vi "Autonomous Independent.vi"   [LabVIEW 2015]
doc: "This VI is called when autonomous begins, and will automatically be terminated when autonomous ends. You can carry out timed or sensor driven robot movement independently without needing to return to the caller."
uses:
  <vilib>/Rock Robotics/WPI/Utilities/WPI_GetSetVariantRefNum.vi
  <vilib>/Rock Robotics/Network Tables/NT Read String.vi
  <vilib>/Rock Robotics/Network Tables/NT Read Number.vi
  <vilib>/Rock Robotics/Network Tables/NT Write Numeric Array.vi
  <vilib>/Rock Robotics/Network Tables/NT Read Boolean.vi
panel:
  # "Be sure to right-click and choose Data Operations>>Make Current Value default if you want to save the array values with the VI"
types:
  T1 = typedef "WPI_JoystickDevRef.ctl" = cluster{"Device":T2}
  T2 = typedef "WPI_JoystickDeviceEnum.ctl" = enum16{"USB 0", "USB 1", "USB 2", "USB 3", "USB 4", "USB 5"}
  T3 = typedef "WPI_EncoderDevRef.ctl" = cluster{"DevStatus":errorcluster, "EncoderIndex":T4, "CounterIndex":T5, "DistancePerCount":dbl, "Decoding Type":T6}
  T4 = typedef "FPGA_EncoderIdx.ctl" = enum8{"Enc 0", "Enc 1", "Enc 2", "Enc 3", "Enc 4", "Enc 5", "Enc 6", "Enc 7", "Invalid"}
  T5 = typedef "FPGA_CounterCtrSystemIndex.ctl" = enum8{"Ctr 0", "Ctr 1", "Ctr 2", "Ctr 3", "Ctr 4", "Ctr 5", "Ctr 6", "Ctr 7", "Invalid"}
  T6 = typedef "WPI_EncoderType.ctl" = enum16{"1x", "2x", "4x"}
  T7 = typedef "WPI_MotorControlDeviceRef.ctl" = cluster{"DeviceStatus":errorcluster, "Type":T8, "PWM":cluster{"PWM Channel":T9, "DeadBand":T10}, "CAN":cluster{"Device Number":u8, "Control Mode":T11, "Semaphore":T12, "Max Vout":dbl, "TalonSRX Control Mode":T13}, "Invert":bool}
  T8 = typedef "WPI_MotorControlType.ctl" = enum16{"PWM", "CAN", "CANTalonSRX"}
  T9 = typedef "FPGA_DIOPWMChannel.ctl" = enum8{"PWM 0", "PWM 1", "PWM 2", "PWM 3", "PWM 4", "PWM 5", "PWM 6", "PWM 7", "PWM 8", "PWM 9", "PWM MXP 0", "PWM MXP 1", "PWM MXP 2", "PWM MXP 3", "PWM MXP 4", "PWM MXP 5", "PWM MXP 6", "PWM MXP 7", "PWM MXP 8", "PWM MXP 9", "Invalid"}
  T10 = typedef "WPI_PWMDeadband.ctl" = cluster{"Name":string, "maxPositivePwm":i32, "minPositivePwm":i32, "centerPwm":i32, "maxNegativePwm":i32, "minNegativePwm":i32, "angularRange":u16}
  T11 = typedef "WPI_CANJaguar_ControlMode.ctl" = enum8{"Percent VBus", "Current", "Speed", "Position", "Voltage"}
  T12 = typedef "Semaphore RefNum" = refnum<k1>
  T13 = typedef "WPI_CANTalonSRX_APIControlMode.ctl" = enum8{"Percent VBus", "Speed", "Position", "Slave", "Unchanged / Invalid", "Voltage Compensation", "Current", "Motion Profile"}
  T14 = typedef "WPI_GyroDevRef.ctl" = cluster{"DevStatus":errorcluster, "Analog Channel":T15, "Offset":dbl, "Gain (VoltsPerDegree/Second)":dbl, "Gyro Type":enum16{"Analog", "XRS450"}, "Handle":i32, "SPI Bus":T16, "Device Found":bool, "Sample Rate":dbl, "Calibrate On Open":bool}
  T15 = typedef "FPGA_AIChannel.ctl" = enum8{"AI 0", "AI 1", "AI 2", "AI 3", "AI MXP 0", "AI MXP 1", "AI MXP 2", "AI MXP 3", "Invalid"}
  T16 = typedef "spi_bus.ctl" = enum16{"SPI On-Board, CS0", "SPI On-Board, CS1", "SPI On-Board, CS2", "SPI On-Board, CS3", "SPI MXP", "Invalid"}
  T17 = typedef "WPI_RobotDriveDevRef.ctl" = cluster{"DevStatus":errorcluster, "Motors[]":T7[], "Square Inputs":bool, "Max Output":dbl}
  T18 = typedef "WPI_DigitalInputDevRef.ctl" = cluster{"DevStatus":errorcluster, "DIO Channel":T19}
  T19 = typedef "FPGA_DIOChannel.ctl" = enum8{"DIO 0", "DIO 1", "DIO 2", "DIO 3", "DIO 4", "DIO 5", "DIO 6", "DIO 7", "DIO 8", "DIO 9", "DIO MXP 0", "DIO MXP 1", "DIO MXP 2", "DIO MXP 3", "DIO MXP 4", "DIO MXP 5", "DIO MXP 6", "DIO MXP 7", "DIO MXP 8", "DIO MXP 9", "DIO MXP 10", "DIO MXP 11", "DIO MXP 12", "DIO MXP 13", "DIO MXP 14", "DIO MXP 15", "Invalid"}
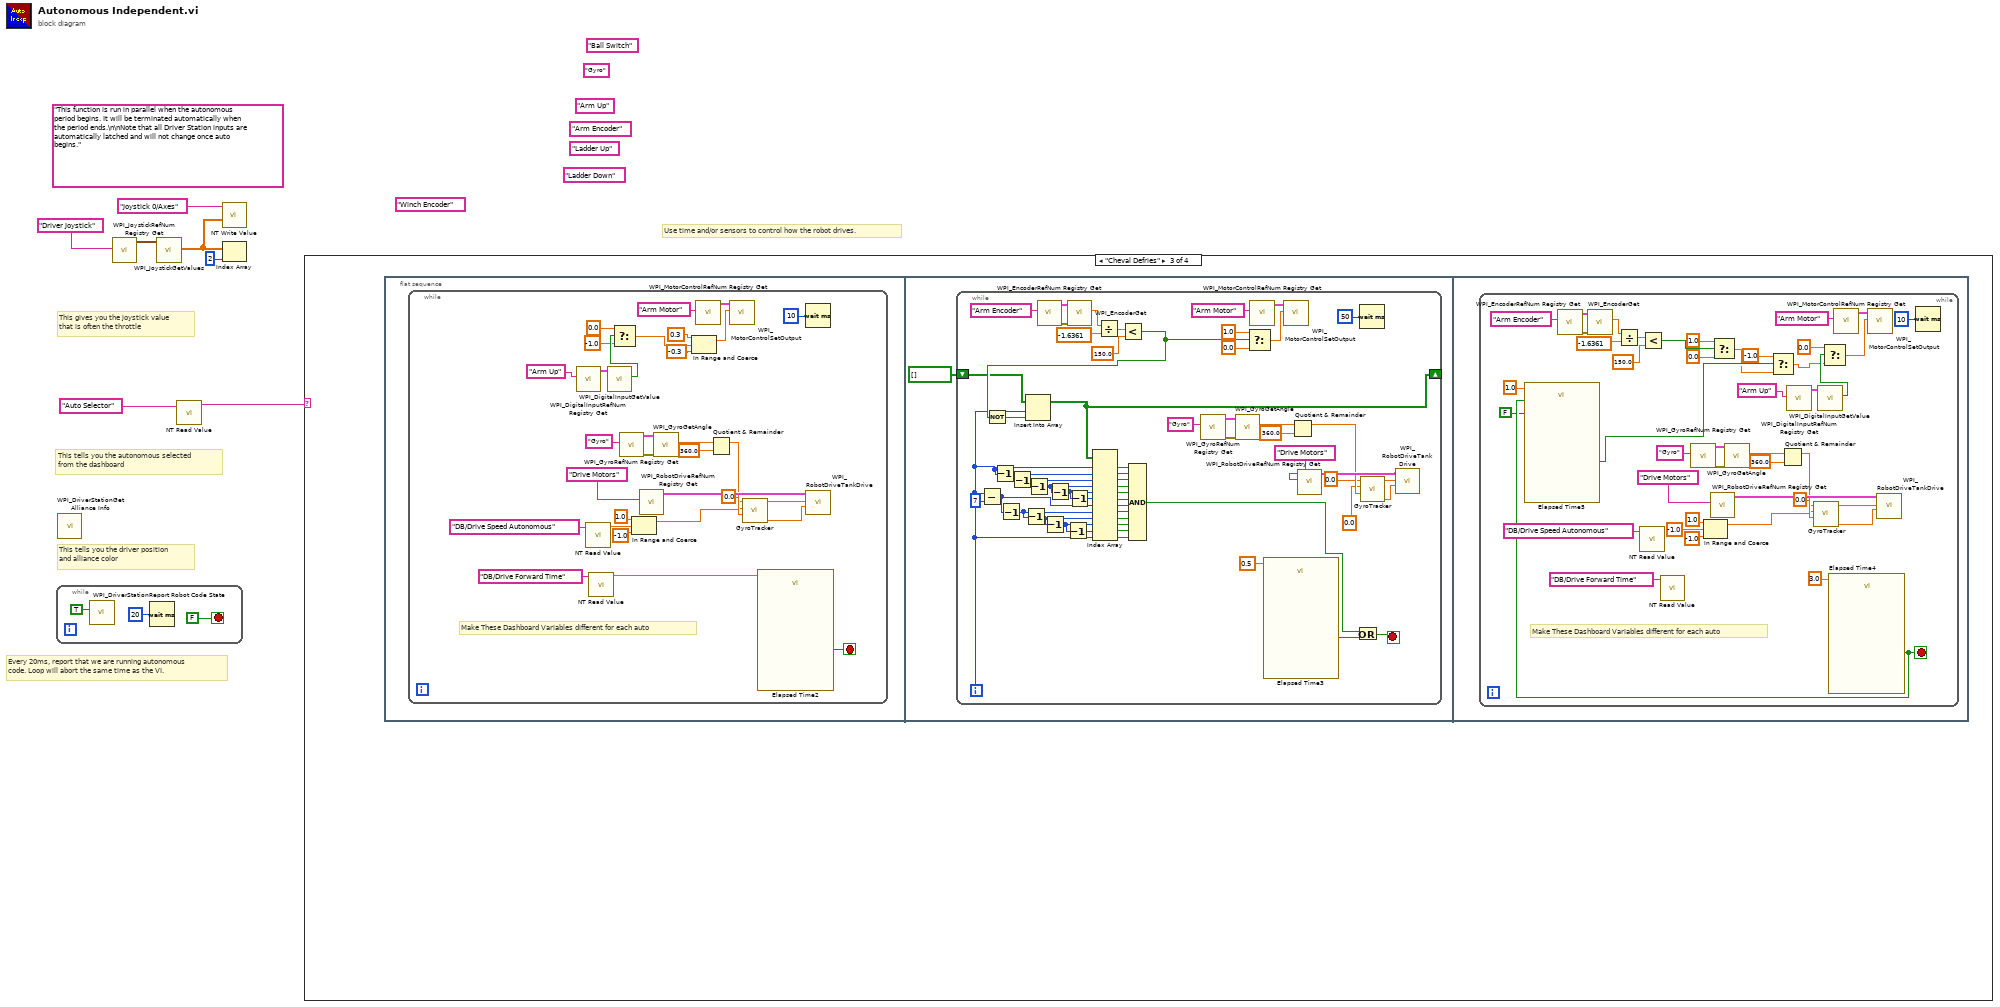
[diagram p0: block diagram]
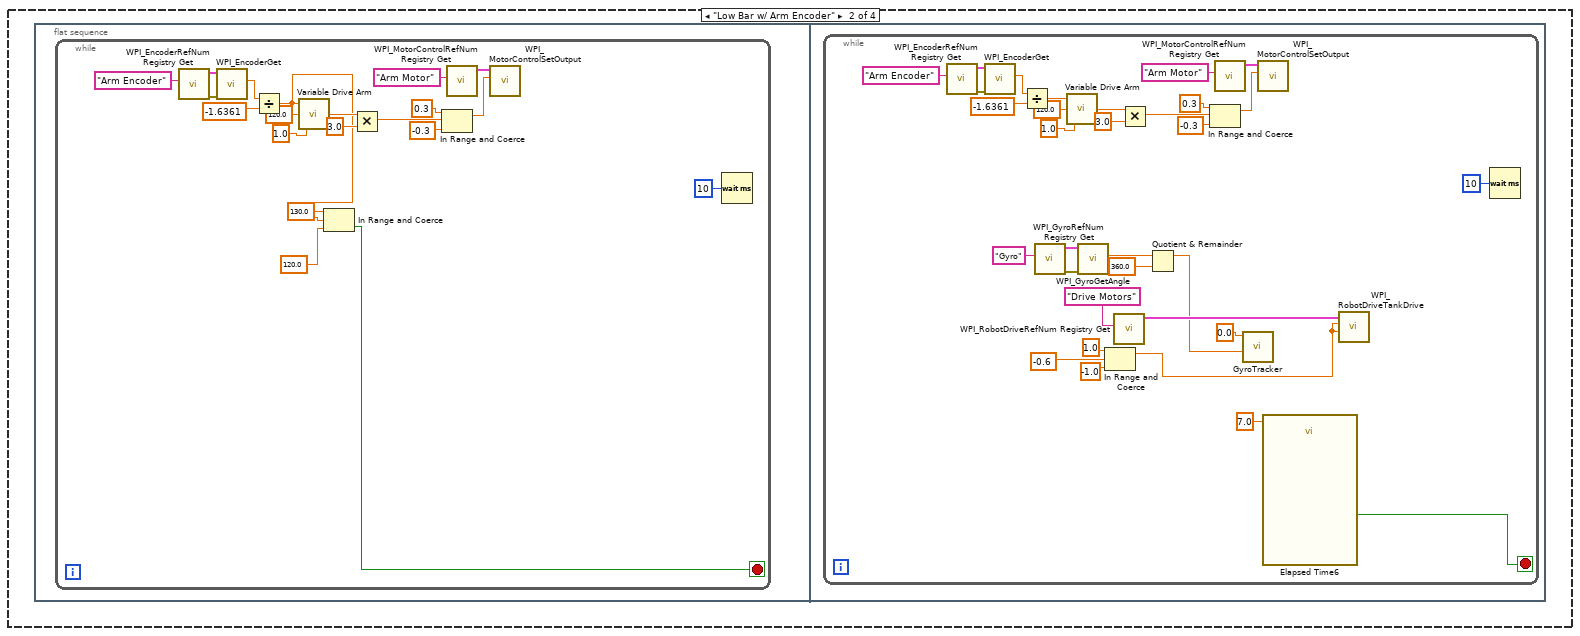
[diagram p3: hidden frame]
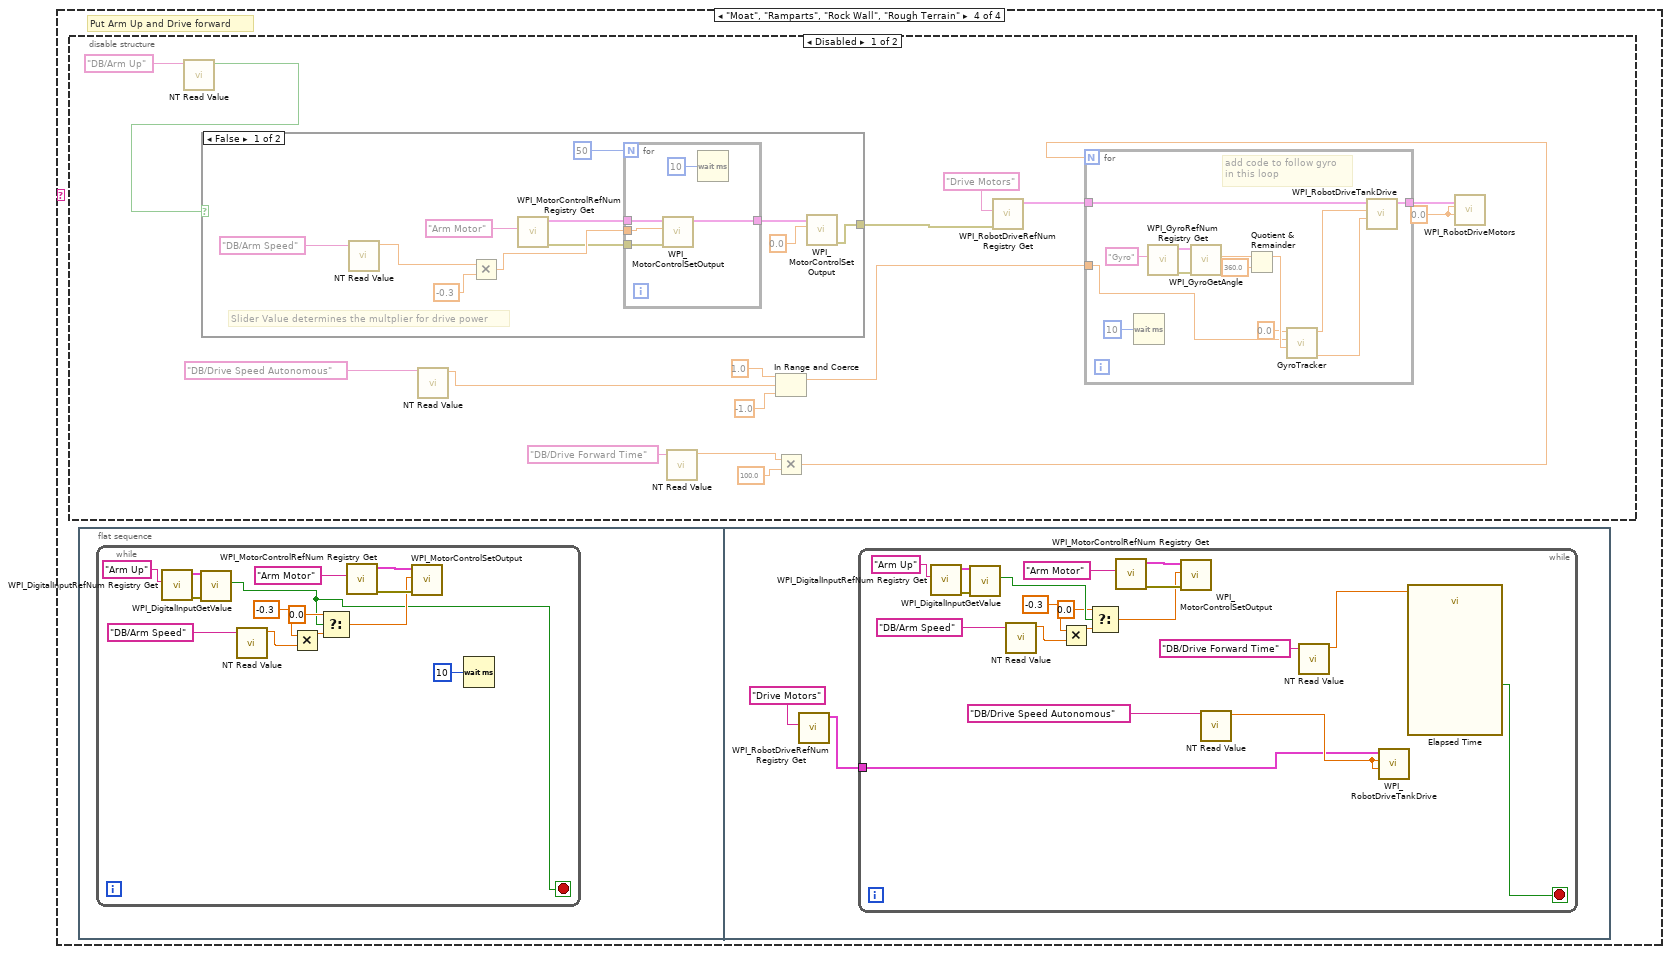
[diagram p4: hidden frame]
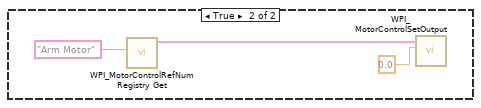
[diagram p5: hidden frame]
diagram:
  (unwired) "Arm Up" ("refnum name")
  (unwired) "Winch Encoder" ("refnum name")
  (unwired) "Ladder Down" ("refnum name")
  (unwired) "Ladder Up" ("refnum name")
  (unwired) "Arm Encoder" ("refnum name")
  (unwired) "Ball Switch" ("refnum name")
  (unwired) "Gyro" ("refnum name")
  (unwired) "This function is run in parallel when the autonomous period begins. It will be terminated automatically when the period ends.\n\nNote that all Driver Station inputs are automatically latched and will not change once auto begins."
  # "This tells you the autonomous selected\nfrom the dashboard"
  # "Every 20ms, report that we are running autonomous\ncode. Loop will abort the same time as the VI."
  # "This gives you the joystick value\nthat is often the throttle"
  # "Use time and/or sensors to control how the robot drives."
  # "This tells you the driver position\nand alliance color"
  n1 = while {
    stop <- FALSE stop-if-true
    n2 = call <vilib>:"WPI_DriverStationReport Robot Code State.vi"("Autonomous"=TRUE) -> ()  [unwired: 10 in, 1 out]
    n3 = Wait (ms)(milliseconds to wait=u32 20) -> ()  [unwired: 1 out]
  }
  n4 = call <vilib>:"WPI_DriverStationGet Alliance Info.vi"() -> ()  [unwired: 12 out]
  n5 = call <vilib>:"WPI_JoystickRefNum Registry Get.vi"("refnum name"="Driver Joystick") -> ("JoystickDevRef"=w6:T1)  [unwired: 1 in, 9 out]
  n6 = call <vilib>:"WPI_JoystickGetValues.vi"("JoystickDevRef"=w6) -> ("Axes"=w2:dbl[])  [unwired: 6 in, 4 out]
  n7 = call-poly <vilib>:"NT Read Value.vi"("Name"="Auto Selector") -> ("String"=w3:string)  [unwired: 9 in, 1 out]
  n8 = call-poly <vilib>:"NT Write Value.vi"("Numeric Array"=w2, "Name"="Joystick 0/Axes") -> ()  [unwired: 9 in, 1 out]
  n9 = Index Array(array=w2, index=2) -> ()  [unwired: 1 out]
  n10 = case shown="\"Cheval Defries\"" w3 {
    frame Default {
      # "You can put your main auto here, or you can right-click on the case and make any\nother frame be the default case."
      # "This is the frame that will execute if no selection is made, or if it is not recognized"
    }
    frame "Low Bar w/ Arm Encoder" {
      n11 = flat-sequence {
        frame #0 {
          n12 = while {
            stop <- w11 stop-if-true
            n13 = call <vilib>:"WPI_EncoderRefNum Registry Get.vi"("refnum name"="Arm Encoder") -> ("error out"=w24:errorcluster, "EncoderDevRef"=w25:T3)  [unwired: 9 in]
            n14 = call <vilib>:"WPI_EncoderGet.vi"("error in (no error)"=w24, "EncoderDevRef"=w25) -> ("Distance"=w26:dbl)  [unwired: 4 in, 5 out]
            n15 = Divide(x=w26, y=-1.6361 ("Arm Calibration")) -> (x/y=w14:dbl)
            n16 = call "Variable Drive Arm.vi"("Max Speed"=1.0, "Wanted Angle"=120.0, "Encoder"=w14) -> ("Motor Controller"=w18:dbl)
            n17 = In Range and Coerce(upper limit=130.0, x=w14, lower limit=120.0) -> (In Range?=w11:bool)  [unwired: 1 out]
            n18 = Multiply(x=w18, y=3.0) -> (x*y=w16:dbl)
            n19 = In Range and Coerce(upper limit=0.3, x=w16, lower limit=-0.3) -> (coerced(x)=w20:dbl)  [unwired: 1 out]
            n20 = call <vilib>:"WPI_MotorControlRefNum Registry Get.vi"("refnum name"="Arm Motor") -> ("MotorControlDevRef"=w21:T7)  [unwired: 9 in, 1 out]
            n21 = call <vilib>:"WPI_MotorControlSetOutput.vi"("Output"=w20, "MotorControlDevRef"=w21) -> ()  [unwired: 7 in, 3 out]
            n22 = Wait (ms)(milliseconds to wait=u32 10) -> ()  [unwired: 1 out]
          }
        }
        frame #1 {
          n23 = while {
            stop <- w62 stop-if-true
            n24 = call <vilib>:"WPI_EncoderRefNum Registry Get.vi"("refnum name"="Arm Encoder") -> ("error out"=w55:errorcluster, "EncoderDevRef"=w56:T3)  [unwired: 9 in]
            n25 = call <vilib>:"WPI_EncoderGet.vi"("error in (no error)"=w55, "EncoderDevRef"=w56) -> ("Distance"=w57:dbl)  [unwired: 4 in, 5 out]
            n26 = Divide(x=w57, y=-1.6361 ("Arm Calibration")) -> (x/y=w54:dbl)
            n27 = call <vilib>:"WPI_GyroRefNum Registry Get.vi"("refnum name"="Gyro") -> ("error out"=w36:errorcluster, "GyroDevRef"=w37:T14)  [unwired: 9 in]
            n28 = call "Variable Drive Arm.vi"("Max Speed"=1.0, "Wanted Angle"=120.0, "Encoder"=w54) -> ("Motor Controller"=w47:dbl)
            n29 = call <vilib>:"WPI_GyroGetAngle.vi"("error in"=w36, "GyroDevRef"=w37) -> ("Angle"=w39:dbl)  [unwired: 5 in, 4 out]
            n30 = In Range and Coerce(upper limit=1.0, x=-0.6, lower limit=-1.0) -> (coerced(x)=w33:dbl)  [unwired: 1 out]
            n31 = call <vilib>:"WPI_RobotDriveRefNum Registry Get.vi"("refnum name"="Drive Motors") -> ("RobotDriveDevRef"=w44:T17)  [unwired: 1 in, 9 out]
            n32 = Multiply(x=w47, y=3.0) -> (x*y=w45:dbl)
            n33 = Quotient & Remainder(x=w39, y=360.0) -> (x-y*floor(x/y)=w35:dbl)  [unwired: 1 out]
            n34 = In Range and Coerce(upper limit=0.3, x=w45, lower limit=-0.3) -> (coerced(x)=w50:dbl)  [unwired: 1 out]
            n35 = call <vilib>:"WPI_MotorControlRefNum Registry Get.vi"("refnum name"="Arm Motor") -> ("MotorControlDevRef"=w51:T7)  [unwired: 9 in, 1 out]
            n36 = call "GyroTracker.vi"("Gyro Angle"=w35, "Target Direction (degrees)"=0.0) -> ()  [unwired: 8 in, 2 out]
            n37 = call <vilib>:"WPI_MotorControlSetOutput.vi"("Output"=w50, "MotorControlDevRef"=w51) -> ()  [unwired: 7 in, 3 out]
            n38 = call "Elapsed Time6"("Time Target (s)"=7.0) -> ("Time has Elapsed"=w62:bool)  [unwired: 11 in, 7 out]
            n39 = call <vilib>:"WPI_RobotDriveTankDrive.vi"("Right axis value"=w33, "Left axis value"=w33, "RobotDriveDevRef"=w44) -> ()  [unwired: 6 in, 3 out]
            n40 = Wait (ms)(milliseconds to wait=u32 10) -> ()  [unwired: 1 out]
          }
        }
      }
    }
    frame "Cheval Defries" {
      n41 = flat-sequence {
        frame #0 {
          n42 = while {
            stop <- w93 stop-if-true
            # "Make These Dashboard Variables different for each auto"
            n43 = call <vilib>:"WPI_DigitalInputRefNum Registry Get.vi"("refnum name"="Arm Up") -> ("DigitalInputDevRef"=w66:T18)  [unwired: 9 in, 1 out]
            n44 = call-poly <vilib>:"NT Read Value.vi"("Name"="DB/Drive Speed Autonomous") -> ("Numeric"=w83:dbl)  [unwired: 9 in, 1 out]
            n45 = call-poly <vilib>:"NT Read Value.vi"("Name"="DB/Drive Forward Time") -> ("Numeric"=w81:dbl)  [unwired: 9 in, 1 out]
            n46 = call <vilib>:"WPI_DigitalInputGetValue.vi"("DigitalInputDevRef"=w66) -> ("Value"=w65:bool)  [unwired: 8 in, 2 out]
            n47 = Select(t=0.0, s=w65, f=-1.0) -> (s? t:f=w63:dbl)
            n48 = call <vilib>:"WPI_GyroRefNum Registry Get.vi"("refnum name"="Gyro") -> ("error out"=w72:errorcluster, "GyroDevRef"=w73:T14)  [unwired: 9 in]
            n49 = In Range and Coerce(upper limit=1.0, x=w83, lower limit=-1.0) -> (coerced(x)=w69:dbl)  [unwired: 1 out]
            n50 = call <vilib>:"WPI_RobotDriveRefNum Registry Get.vi"("refnum name"="Drive Motors") -> ("RobotDriveDevRef"=w79:T17)  [unwired: 1 in, 9 out]
            n51 = call <vilib>:"WPI_GyroGetAngle.vi"("error in"=w72, "GyroDevRef"=w73) -> ("Angle"=w75:dbl)  [unwired: 5 in, 4 out]
            n52 = In Range and Coerce(upper limit=0.3, x=w63, lower limit=-0.3) -> (coerced(x)=w88:dbl)  [unwired: 1 out]
            n53 = call <vilib>:"WPI_MotorControlRefNum Registry Get.vi"("refnum name"="Arm Motor") -> ("MotorControlDevRef"=w89:T7)  [unwired: 9 in, 1 out]
            n54 = Quotient & Remainder(x=w75, y=360.0) -> (x-y*floor(x/y)=w71:dbl)  [unwired: 1 out]
            n55 = call <vilib>:"WPI_MotorControlSetOutput.vi"("Output"=w88, "MotorControlDevRef"=w89) -> ()  [unwired: 7 in, 3 out]
            n56 = call "GyroTracker.vi"("Gyro Angle"=w71, "Target Speed"=w69, "Target Direction (degrees)"=0.0) -> ("Right Wheel Speed"=w77:dbl, "Left Wheel Speed"=w78:dbl)  [unwired: 7 in]
            n57 = call "Elapsed Time2"("Time Target (s)"=w81) -> ("Time has Elapsed"=w93:bool)  [unwired: 11 in, 7 out]
            n58 = Wait (ms)(milliseconds to wait=u32 10) -> ()  [unwired: 1 out]
            n59 = call <vilib>:"WPI_RobotDriveTankDrive.vi"("Right axis value"=w77, "Left axis value"=w78, "RobotDriveDevRef"=w79) -> ()  [unwired: 6 in, 3 out]
          }
        }
        frame #1 {
          n60 = while {
            shift-right: [w99] -> _
            shift-left: bool[] [] -> [w100]
            i -> [w98]
            stop <- w103 stop-if-true
            n61 = Subtract(x=w98, y=7) -> (x-y=w120:i32)
            n62 = Decrement(x=w98) -> (x-1=w123:i32)
            n63 = Decrement(x=w120) -> (x-1=w119:i32)
            n64 = Decrement(x=w123) -> (x-1=w125:i32)
            n65 = Decrement(x=w119) -> (x-1=w118:i32)
            n66 = Decrement(x=w125) -> (x-1=w127:i32)
            n67 = call <vilib>:"WPI_EncoderRefNum Registry Get.vi"("refnum name"="Arm Encoder") -> ("error out"=w133:errorcluster, "EncoderDevRef"=w134:T3)  [unwired: 9 in]
            n68 = Decrement(x=w118) -> (x-1=w116:i32)
            n69 = Decrement(x=w127) -> (x-1=w124:i32)
            n70 = Decrement(x=w116) -> (x-1=w117:i32)
            n71 = call <vilib>:"WPI_EncoderGet.vi"("error in (no error)"=w133, "EncoderDevRef"=w134) -> ("Distance"=w135:dbl)  [unwired: 4 in, 5 out]
            n72 = Decrement(x=w124) -> (x-1=w126:i32)
            n73 = Divide(x=w135, y=-1.6361 ("Arm Calibration")) -> (x/y=w128:dbl)
            n74 = Less?(x=w128, y=150.0) -> (x < y?=w101:bool)
            n75 = Not(x=w101) -> (.not. x?=w95:bool)
            n76 = Insert Into Array(array=w100, index=w98, new element=w95) -> (w99:bool[])
            n77 = Index Array(array=w99, index #1=w98, index #2=w123, index #3=w125, index #4=w127, index #5=w124, index #6=w126, index #7=w120, index #8=w119, index #9=w118, index #10=w116, index #11=w117, index #12=w98) -> (element #1=w115:bool, element #2=w114:bool, element #3=w113:bool, element #4=w112:bool, element #5=w111:bool, element #6=w110:bool, element #7=w109:bool, element #8=w108:bool, element #9=w107:bool, element #10=w106:bool, element #11=w105:bool, element #12=w97:bool)
            n78 = Compound Arithmetic op=AND(w115, w114, w113, w112, w111, w110, w109, w108, w107, w106, w105, w97) -> (w96:bool)
            n79 = call <vilib>:"WPI_GyroRefNum Registry Get.vi"("refnum name"="Gyro") -> ("error out"=w141:errorcluster, "GyroDevRef"=w142:T14)  [unwired: 9 in]
            n80 = call <vilib>:"WPI_GyroGetAngle.vi"("error in"=w141, "GyroDevRef"=w142) -> ("Angle"=w144:dbl)  [unwired: 5 in, 4 out]
            n81 = Select(t=1.0, s=w101, f=0.0) -> (s? t:f=w131:dbl)
            n82 = call <vilib>:"WPI_MotorControlRefNum Registry Get.vi"("refnum name"="Arm Motor") -> ("MotorControlDevRef"=w150:T7)  [unwired: 9 in, 1 out]
            n83 = call "Elapsed Time3"("Time Target (s)"=0.5) -> ("Time has Elapsed"=w104:bool)  [unwired: 11 in, 7 out]
            n84 = call <vilib>:"WPI_MotorControlSetOutput.vi"("Output"=w131, "MotorControlDevRef"=w150) -> ()  [unwired: 7 in, 3 out]
            n85 = Quotient & Remainder(x=w144, y=360.0) -> (x-y*floor(x/y)=w140:dbl)  [unwired: 1 out]
            n86 = call <vilib>:"WPI_RobotDriveRefNum Registry Get.vi"("refnum name"="Drive Motors") -> ("RobotDriveDevRef"=w147:T17)  [unwired: 1 in, 9 out]
            n87 = Or(x=w96, y=w104) -> (x .or. y?=w103:bool)
            n88 = Wait (ms)(milliseconds to wait=u32 50) -> ()  [unwired: 1 out]
            n89 = call "GyroTracker.vi"("Gyro Angle"=w140, "Target Speed"=0.0, "Target Direction (degrees)"=0.0) -> ("Right Wheel Speed"=w122:dbl, "Left Wheel Speed"=w146:dbl)  [unwired: 7 in]
            n90 = call <vilib>:"WPI_RobotDriveTankDrive.vi"("Right axis value"=w122, "Left axis value"=w146, "RobotDriveDevRef"=w147) -> ()  [unwired: 6 in, 3 out]
          }
        }
        frame #2 {
          n91 = while {
            stop <- w165 stop-if-true
            # "Make These Dashboard Variables different for each auto"
            n92 = call <vilib>:"WPI_EncoderRefNum Registry Get.vi"("refnum name"="Arm Encoder") -> ("error out"=w172:errorcluster, "EncoderDevRef"=w173:T3)  [unwired: 9 in]
            n93 = call <vilib>:"WPI_EncoderGet.vi"("error in (no error)"=w172, "EncoderDevRef"=w173) -> ("Distance"=w174:dbl)  [unwired: 4 in, 5 out]
            n94 = Divide(x=w174, y=-1.6361 ("Arm Calibration")) -> (x/y=w168:dbl)
            n95 = call-poly <vilib>:"NT Read Value.vi"("Name"="DB/Drive Speed Autonomous") -> ()  [unwired: 9 in, 2 out]
            n96 = Less?(x=w168, y=150.0) -> (x < y?=w167:bool)
            n97 = call-poly <vilib>:"NT Read Value.vi"("Name"="DB/Drive Forward Time") -> ()  [unwired: 9 in, 2 out]
            n98 = call <vilib>:"WPI_GyroRefNum Registry Get.vi"("refnum name"="Gyro") -> ("error out"=w181:errorcluster, "GyroDevRef"=w182:T14)  [unwired: 9 in]
            n99 = In Range and Coerce(upper limit=1.0, x=-1.0, lower limit=-1.0) -> (coerced(x)=w178:dbl)  [unwired: 1 out]
            n100 = call <vilib>:"WPI_RobotDriveRefNum Registry Get.vi"("refnum name"="Drive Motors") -> ("RobotDriveDevRef"=w188:T17)  [unwired: 1 in, 9 out]
            n101 = Select(t=1.0, s=w167, f=0.0) -> (s? t:f=w161:dbl)
            n102 = call <vilib>:"WPI_GyroGetAngle.vi"("error in"=w181, "GyroDevRef"=w182) -> ("Angle"=w184:dbl)  [unwired: 5 in, 4 out]
            n103 = Quotient & Remainder(x=w184, y=360.0) -> (x-y*floor(x/y)=w180:dbl)  [unwired: 1 out]
            n104 = call <vilib>:"WPI_DigitalInputRefNum Registry Get.vi"("refnum name"="Arm Up") -> ("DigitalInputDevRef"=w152:T18)  [unwired: 9 in, 1 out]
            n105 = call "GyroTracker.vi"("Gyro Angle"=w180, "Target Speed"=w178, "Target Direction (degrees)"=0.0) -> ("Right Wheel Speed"=w186:dbl, "Left Wheel Speed"=w187:dbl)  [unwired: 7 in]
            n106 = call <vilib>:"WPI_DigitalInputGetValue.vi"("DigitalInputDevRef"=w152) -> ("Value"=w155:bool)  [unwired: 8 in, 2 out]
            n107 = call "Elapsed Time4"("Time Target (s)"=3.0) -> ("Time has Elapsed"=w165:bool)  [unwired: 11 in, 7 out]
            n108 = call "Elapsed Time5"("Time Target (s)"=1.0, "Reset"=w165, "Auto Reset"=FALSE) -> ("Time has Elapsed"=w163:bool)  [unwired: 9 in, 7 out]
            n109 = Select(t=-1.0, s=w163, f=w161) -> (s? t:f=w154:dbl)
            n110 = Select(t=0.0, s=w155, f=w154) -> (s? t:f=w156:dbl)
            n111 = call <vilib>:"WPI_MotorControlRefNum Registry Get.vi"("refnum name"="Arm Motor") -> ("MotorControlDevRef"=w177:T7)  [unwired: 9 in, 1 out]
            n112 = call <vilib>:"WPI_MotorControlSetOutput.vi"("Output"=w156, "MotorControlDevRef"=w177) -> ()  [unwired: 7 in, 3 out]
            n113 = call <vilib>:"WPI_RobotDriveTankDrive.vi"("Right axis value"=w186, "Left axis value"=w187, "RobotDriveDevRef"=w188) -> ()  [unwired: 6 in, 3 out]
            n114 = Wait (ms)(milliseconds to wait=u32 10) -> ()  [unwired: 1 out]
          }
        }
      }
    }
    frame "Moat", "Ramparts", "Rock Wall", "Rough Terrain" {
      # "Put Arm Up and Drive forward"
      n115 = disable-structure shown="Disabled" {
        frame Disabled {
          w207 = 0.0 ("Y axis value")
          n116 = call-poly <vilib>:"NT Read Value.vi"("Name"="DB/Arm Up") -> ("Boolean"=w200:bool)  [unwired: 9 in, 1 out]
          n117 = case shown="False" w200 {
            tunnel: [w211 _] -> w201
            frame False {
              # "Slider Value determines the multplier for drive power"
              n118 = call-poly <vilib>:"NT Read Value.vi"("Name"="DB/Arm Speed") -> ("Numeric"=w216:dbl)  [unwired: 9 in, 1 out]
              n119 = Multiply(x=w216, y=-0.3) -> (x*y=w221:dbl)
              n120 = call <vilib>:"WPI_MotorControlRefNum Registry Get.vi"("refnum name"="Arm Motor") -> ("error out"=w220:errorcluster, "MotorControlDevRef"=w219:T7)  [unwired: 9 in]
              n121 = for {
                N: 50 -> [_]
                tunnel: w219 -> [w225]
                tunnel: w220 -> [w224]
                tunnel: w221 -> [w223]
                tunnel: [w222] -> w212
                n122 = call <vilib>:"WPI_MotorControlSetOutput.vi"("error in (no error)"=w224, "Output"=w223, "MotorControlDevRef"=w225) -> ("MotorControlDevRef"=w222:T7)  [unwired: 6 in, 2 out]
                n123 = Wait (ms)(milliseconds to wait=u32 10) -> ()  [unwired: 1 out]
              }
              n124 = call <vilib>:"WPI_MotorControlSetOutput.vi"("Output"=0.0, "MotorControlDevRef"=w212) -> ("error out"=w211:errorcluster)  [unwired: 7 in, 2 out]
            }
            frame True {
              n125 = call <vilib>:"WPI_MotorControlRefNum Registry Get.vi"("refnum name"="Arm Motor") -> ("MotorControlDevRef"=w228:T7)  [unwired: 9 in, 1 out]
              n126 = call <vilib>:"WPI_MotorControlSetOutput.vi"("Output"=0.0, "MotorControlDevRef"=w228) -> ()  [unwired: 7 in, 3 out]
            }
          }
          n127 = call-poly <vilib>:"NT Read Value.vi"("Name"="DB/Drive Speed Autonomous") -> ("Numeric"=w205:dbl)  [unwired: 9 in, 1 out]
          n128 = call-poly <vilib>:"NT Read Value.vi"("Name"="DB/Drive Forward Time") -> ("Numeric"=w196:dbl)  [unwired: 9 in, 1 out]
          n129 = In Range and Coerce(upper limit=1.0, x=w205, lower limit=-1.0) -> (coerced(x)=w199:dbl)  [unwired: 1 out]
          n130 = Multiply(x=w196, y=100.0) -> (x*y=w198:dbl)
          n131 = call <vilib>:"WPI_RobotDriveRefNum Registry Get.vi"("error in (no error)"=w201, "refnum name"="Drive Motors") -> ("RobotDriveDevRef"=w209:T17)  [unwired: 9 out]
          n132 = for {
            N: w198 -> [_]
            tunnel: w209 -> [w232]
            tunnel: w199 -> [w230]
            tunnel: [w231] -> w208
            # "add code to follow gyro\nin this loop"
            n133 = Wait (ms)(milliseconds to wait=u32 10) -> ()  [unwired: 1 out]
            n134 = call <vilib>:"WPI_GyroRefNum Registry Get.vi"("refnum name"="Gyro") -> ("error out"=w235:errorcluster, "GyroDevRef"=w236:T14)  [unwired: 9 in]
            n135 = call <vilib>:"WPI_GyroGetAngle.vi"("error in"=w235, "GyroDevRef"=w236) -> ("Angle"=w238:dbl)  [unwired: 5 in, 4 out]
            n136 = Quotient & Remainder(x=w238, y=360.0) -> (x-y*floor(x/y)=w234:dbl)  [unwired: 1 out]
            n137 = call "GyroTracker.vi"("Gyro Angle"=w234, "Target Speed"=w230, "Target Direction (degrees)"=0.0) -> ("Right Wheel Speed"=w240:dbl, "Left Wheel Speed"=w241:dbl)  [unwired: 7 in]
            n138 = call <vilib>:"WPI_RobotDriveTankDrive.vi"("Right axis value"=w240, "Left axis value"=w241, "RobotDriveDevRef"=w232) -> ("RobotDriveDevRef"=w231:T17)  [unwired: 6 in, 2 out]
          }
          n139 = call <vilib>:"WPI_RobotDriveMotors.vi"("RightSpeed"=w207, "LeftSpeed"=w207, "RobotDriveDevRef"=w208) -> ()  [unwired: 6 in, 3 out]
        }
        frame Enabled {
        }
      }
      n140 = flat-sequence {
        frame #0 {
          n141 = while {
            stop <- w244 stop-if-true
            n142 = call <vilib>:"WPI_DigitalInputRefNum Registry Get.vi"("refnum name"="Arm Up") -> ("error out"=w255:errorcluster, "DigitalInputDevRef"=w254:T18)  [unwired: 9 in]
            n143 = call <vilib>:"WPI_DigitalInputGetValue.vi"("error in (no error)"=w255, "DigitalInputDevRef"=w254) -> ("Value"=w244:bool)  [unwired: 7 in, 2 out]
            n144 = call-poly <vilib>:"NT Read Value.vi"("Name"="DB/Arm Speed") -> ("Numeric"=w249:dbl)  [unwired: 9 in, 1 out]
            n145 = Multiply(x=-0.3 ("Numeric"), y=w249) -> (x*y=w248:dbl)
            n146 = Select(t=0.0, s=w244, f=w248) -> (s? t:f=w245:dbl)
            n147 = call <vilib>:"WPI_MotorControlRefNum Registry Get.vi"("refnum name"="Arm Motor") -> ("error out"=w251:errorcluster, "MotorControlDevRef"=w252:T7)  [unwired: 9 in]
            n148 = call <vilib>:"WPI_MotorControlSetOutput.vi"("error in (no error)"=w251, "Output"=w245, "MotorControlDevRef"=w252) -> ()  [unwired: 6 in, 3 out]
            n149 = Wait (ms)(milliseconds to wait=u32 10) -> ()  [unwired: 1 out]
          }
        }
        frame #1 {
          n150 = call <vilib>:"WPI_RobotDriveRefNum Registry Get.vi"("refnum name"="Drive Motors") -> ("RobotDriveDevRef"=w257:T17)  [unwired: 1 in, 9 out]
          n151 = while {
            tunnel: w257 -> [w259]
            stop <- w261 stop-if-true
            n152 = call <vilib>:"WPI_DigitalInputRefNum Registry Get.vi"("refnum name"="Arm Up") -> ("error out"=w276:errorcluster, "DigitalInputDevRef"=w275:T18)  [unwired: 9 in]
            n153 = call <vilib>:"WPI_DigitalInputGetValue.vi"("error in (no error)"=w276, "DigitalInputDevRef"=w275) -> ("Value"=w267:bool)  [unwired: 7 in, 2 out]
            n154 = call-poly <vilib>:"NT Read Value.vi"("Name"="DB/Arm Speed") -> ("Numeric"=w270:dbl)  [unwired: 9 in, 1 out]
            n155 = Multiply(x=-0.3 ("Numeric"), y=w270) -> (x*y=w269:dbl)
            n156 = Select(t=0.0, s=w267, f=w269) -> (s? t:f=w265:dbl)
            n157 = call <vilib>:"WPI_MotorControlRefNum Registry Get.vi"("refnum name"="Arm Motor") -> ("error out"=w272:errorcluster, "MotorControlDevRef"=w273:T7)  [unwired: 9 in]
            n158 = call <vilib>:"WPI_MotorControlSetOutput.vi"("error in (no error)"=w272, "Output"=w265, "MotorControlDevRef"=w273) -> ()  [unwired: 6 in, 3 out]
            n159 = call-poly <vilib>:"NT Read Value.vi"("Name"="DB/Drive Speed Autonomous") -> ("Numeric"=w260:dbl)  [unwired: 9 in, 1 out]
            n160 = call-poly <vilib>:"NT Read Value.vi"("Name"="DB/Drive Forward Time") -> ("Numeric"=w262:dbl)  [unwired: 9 in, 1 out]
            n161 = call <vilib>:"WPI_RobotDriveTankDrive.vi"("Right axis value"=w260, "Left axis value"=w260, "RobotDriveDevRef"=w259) -> ()  [unwired: 6 in, 3 out]
            n162 = call "Elapsed Time"("Time Target (s)"=w262) -> ("Time has Elapsed"=w261:bool)  [unwired: 11 in, 7 out]
          }
        }
      }
    }
  }
